vi "Read ini Var Keys.vi"(8 "error in (no error)":errorcluster, 10 "section":string, 11 "Base Path":path) -> (0 "error out":errorcluster, 2 "Array":string[](array[string]), 3 "file path":path)   [LabVIEW 2014]
uses:
  <vilib>/Utility/config.llb/NI_LVConfig.lvlib
  <vilib>/Utility/config.llb/Read Key (String).vi
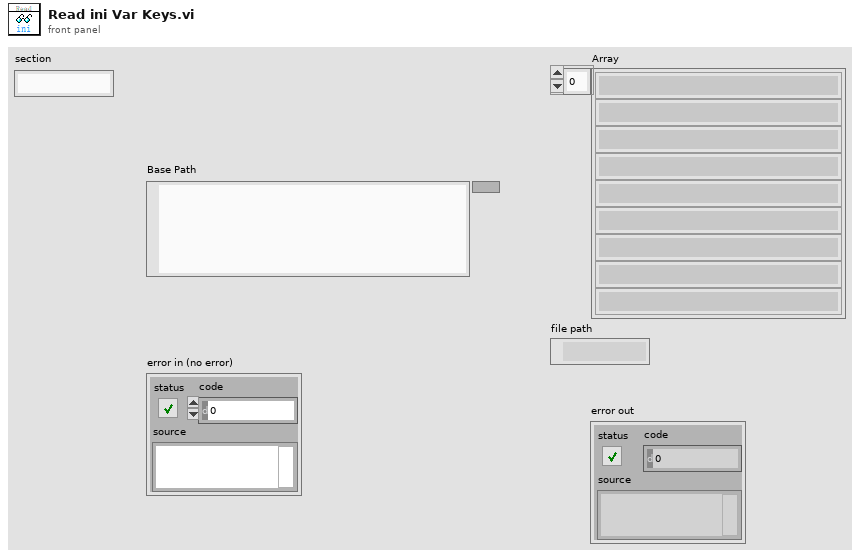
[diagram p1: front panel]
types:
  T1 = typedef "NI_LVConfig.lvlib/Config Data RefNum.ctl" = refnum<k1>
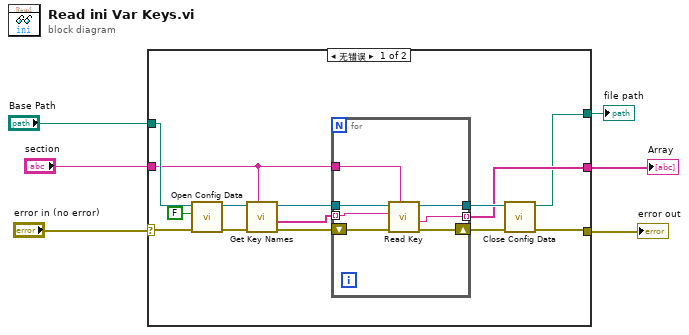
[diagram p0: block diagram]
diagram:
  n1 = case shown="无错误" "error in (no error)" {
    selector: "error in (no error)" -> [w20 w29]
    tunnel: "Base Path" -> [w19 w28]
    tunnel: "section" -> [w14 _]
    tunnel: [w10 w29] -> w3
    tunnel: [w9 _] -> w2
    tunnel: [w8 w28] -> w1
    frame No Error {
      n2 = call <vilib>:"Open Config Data.vi"("error in (no error)"=w20, "create file if necessary (T)"=FALSE, "configuration file path"=w19) -> ("error out"=w18:errorcluster, "refnum"=w17:T1)  [unwired: 6 in, 1 out]
      n3 = call <vilib>:"Get Key Names.vi"("section"=w14, "error in (no error)"=w18, "refnum"=w17) -> ("error out"=w16:errorcluster, "key names"=w13:string[], "refnum out"=w15:T1)  [unwired: 5 in, 1 out]
      n4 = for {
        tunnel: w15 -> [w26]
        tunnel: w14 -> [w25]
        tunnel: w13 -> [w24] mode=indexing
        shift-right: [w23] -> w12
        shift-left: w16 -> [w27]
        tunnel: [w22] -> w11
        tunnel: [w21] -> w9 mode=indexing
        n5 = call-poly <vilib>:"Read Key.vi"("section"=w25, "error in (no error)"=w27, "key"=w24, "refnum"=w26) -> ("error out"=w23:errorcluster, "value"=w21:string, "refnum out"=w22:T1)  [unwired: 4 in, 1 out]
      }
      n6 = call <vilib>:"Close Config Data.vi"("error in (no error)"=w12, "refnum"=w11) -> ("error out"=w10:errorcluster, "file path"=w8:path)  [unwired: 8 in]
    }
    frame Error {
    }
  }
  "error out" <- w3
  "Array" <- w2
  "file path" <- w1
